vi "ring.vi"(11 "input":u16(ring) items=["x2", "x3"]) -> ()   [LabVIEW 2020]
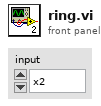
[diagram p1: front panel]
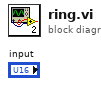
[diagram p0: block diagram]
diagram:
